vi "Lower_Stop_ms1.vi"(8 "error in (no error)":errorcluster, 10 "I-O in":refnum<class "I-O.lvclass">, 11 "Motion in":refnum<class "Motion.lvclass">) -> (0 "error out":errorcluster, 2 "I-O out":refnum<class "I-O.lvclass">, 3 "Motion out":refnum<class "Motion.lvclass">)   [LabVIEW 2016]
uses:
  Classes/Controller/Motion/Motion Folder/Motion.lvclass
  Classes/Controller/I-O/I-O Folder/I-O.lvclass
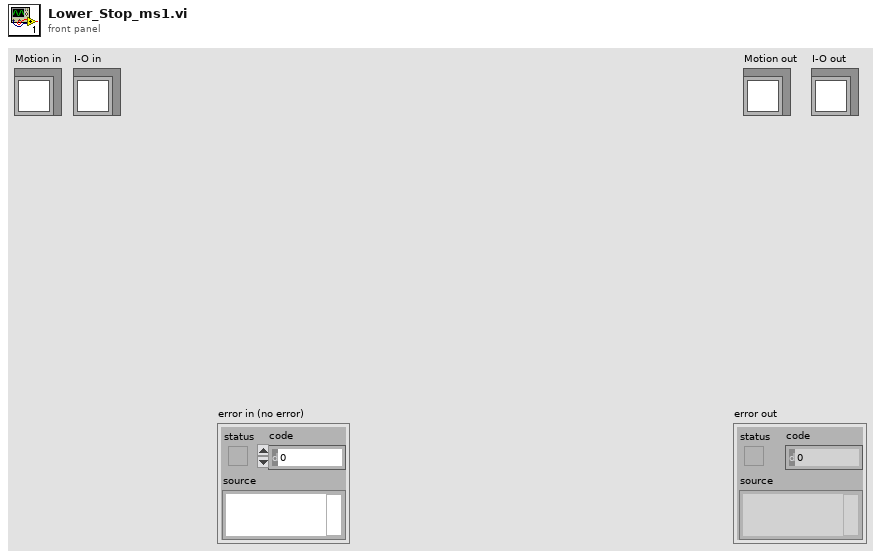
[diagram p1: front panel]
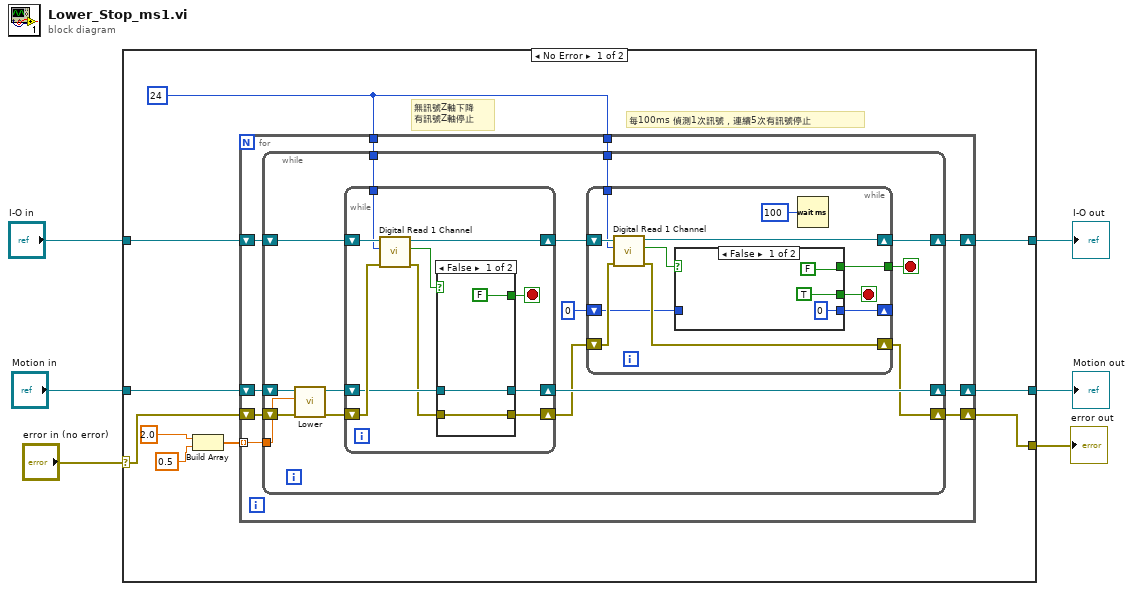
[diagram p0: block diagram]
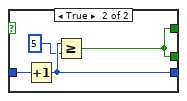
[diagram p2: hidden frame]
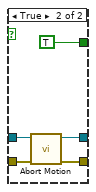
[diagram p3: hidden frame]
diagram:
  n1 = case shown="No Error" "error in (no error)" {
    selector: "error in (no error)" -> [w14 w79]
    tunnel: [w9 w79] -> w5
    tunnel: "Motion in" -> [w16 w78]
    tunnel: "I-O in" -> [w15 w77]
    tunnel: [w8 w78] -> w2
    tunnel: [w7 w77] -> w1
    frame No Error {
      w13 = 24 ("Read")
      # "每100ms 偵測1次訊號，連續5次有訊號停止"
      # "無訊號Z軸下降\n有訊號Z軸停止"
      n2 = Build Array(2.0 ("Speed"), 0.5 ("Speed")) -> (w10:dbl[])
      n3 = for {
        shift-right: [w19] -> w8
        shift-left: w16 -> [w25]
        shift-right: [w22] -> w7
        shift-left: w15 -> [w24]
        shift-right: [w18] -> w9
        shift-left: w14 -> [w23]
        tunnel: w13 -> [w21]
        tunnel: w13 -> [w20]
        tunnel: w10 -> [w17] mode=indexing
        n4 = while {
          tunnel: w21 -> [w33]
          tunnel: w20 -> [w32]
          tunnel: w17 -> [w29]
          shift-right: [w31] -> w19
          shift-left: w25 -> [w40]
          shift-right: [w34] -> w22
          shift-left: w24 -> [w39]
          shift-right: [w30] -> w18
          shift-left: w23 -> [w36]
          stop <- w27 stop-if-true
          n5 = call-dynamic "Lower.vi"("error in (no error)"=w36, "Speed"=w29, "Motion in"=w40) -> ("error out"=w38:errorcluster, "Motion out"=w37:refnum<class "Motion.lvclass">)  [unwired: 7 in]
          n6 = while {
            shift-right: [w63] -> w31
            shift-left: w37 -> [w66]
            shift-right: [w61] -> w35
            shift-left: w39 -> [w68]
            shift-right: [w60] -> w26
            shift-left: w38 -> [w67]
            tunnel: w32 -> [w59]
            stop <- w62 stop-if-true
            n7 = call-dynamic "Digital Read 1 Channel.vi"("error in (no error)"=w67, "Read"=w59, "I-O in"=w68) -> ("error out"=w64:errorcluster, "Value"=w65:bool, "I-O out"=w61:refnum<class "I-O.lvclass">)  [unwired: 6 in]
            n8 = case shown="False" w65 {
              tunnel: w66 -> [w71 w76]
              tunnel: w64 -> [w70 w75]
              tunnel: [w71 w74] -> w63
              tunnel: [w70 w73] -> w60
              tunnel: [FALSE ("Value") TRUE ("Value")] -> w62
              frame False {
              }
              frame True {
                n9 = call-dynamic "Abort Motion.vi"("error in (no error)"=w75, "Motion in"=w76) -> ("error out"=w73:errorcluster, "Motion out"=w74:refnum<class "Motion.lvclass">)  [unwired: 8 in]
              }
            }
          }
          n10 = while {
            shift-right: [w49] -> w34
            shift-left: w35 -> [w50]
            tunnel: w33 -> [w47]
            shift-right: [w45] -> w30
            shift-left: w26 -> [w46]
            shift-right: [w42] -> _
            shift-left: 0 -> [w43]
            tunnel: [w41] -> w27
            stop <- w44 stop-if-true
            n11 = call-dynamic "Digital Read 1 Channel.vi"("error in (no error)"=w46, "Read"=w47, "I-O in"=w50) -> ("error out"=w45:errorcluster, "Value"=w48:bool, "I-O out"=w49:refnum<class "I-O.lvclass">)  [unwired: 6 in]
            n12 = case shown="False" w48 {
              tunnel: [TRUE ("Value") w56] -> w44
              tunnel: w43 -> [_ w58]
              tunnel: [0 w57] -> w42
              tunnel: [FALSE ("Value") w56] -> w41
              frame False {
              }
              frame True {
                n13 = Increment(x=w58) -> (x+1=w57:i32)
                n14 = Greater Or Equal?(x=w57, y=5) -> (x >= y?=w56:bool)
              }
            }
            n15 = Wait (ms)(milliseconds to wait=u32 100) -> ()  [unwired: 1 out]
          }
        }
      }
    }
    frame Error {
    }
  }
  "error out" <- w5
  "Motion out" <- w2
  "I-O out" <- w1
